vi "Configure Step Mode.vi"(0 "VISA resource name":refnum<visa-resource-name>, 1 "Step Frequency (50 Hz)":dbl=50.0 min=43.0 max=1200.0 format="%.2g", 2 "Step Voltage":T1 {"DC Voltage Step Level (0 V)" format="%.3g"; "AC Voltage Step Level (0 V)" format="%.3g"; "DC Voltage (0 V)" format="%.3g"; "AC Voltage (0 V)" format="%.3g"}, 5 "Frequency Step Level (0 Hz)":dbl format="%.1f", 7 "Step Time (1 s)":u32=1 min=1 max=100000, 9 "Step Count (1)":u32=1 min=1 max=99, 11 "error in (no error)":errorcluster, 12 "Step Sync (0: Immediate)":i32(ring) items=["Immediate", "Phase"], 13 "Step Phase (0.0 degrees)":dbl min=0.0 max=359.7 format="%.1f") -> (4 "VISA resource name out":refnum<visa-resource-name>, 15 "error out":errorcluster)   [LabVIEW 2015, in "BK Precision 983X Series.lvlib"]
doc: "Configures all the parameters for step mode.\n\nNote: Run <b>Configure Output Mode.vi</b> first to set the instrument to Step Mode before running this vi."
uses:
  <instrlib>/BK Precision 983X Series/BK Precision 983X Series.lvlib
panel:
  # "degree"
  # "Hz"
  # "V"
  # "V"
  # "V"
  # "V"
  # "s"
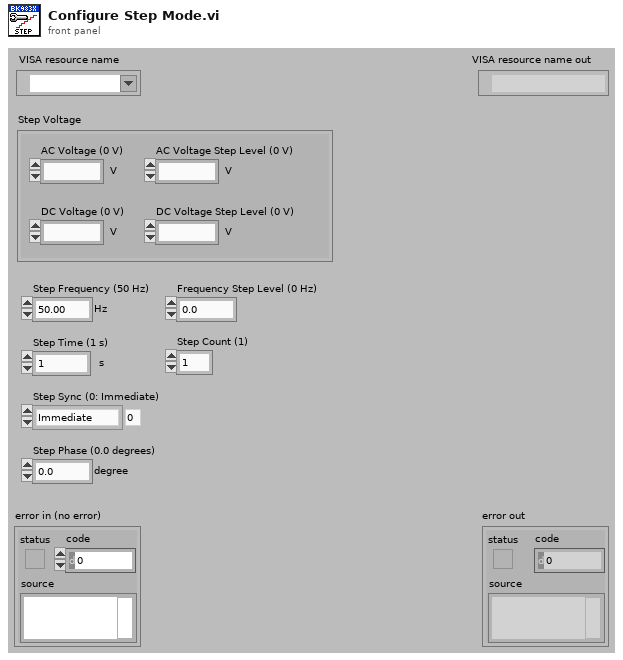
[diagram p1: front panel]
types:
  T1 = cluster{"AC Voltage (0 V)":dbl, "DC Voltage (0 V)":dbl, "AC Voltage Step Level (0 V)":dbl, "DC Voltage Step Level (0 V)":dbl}
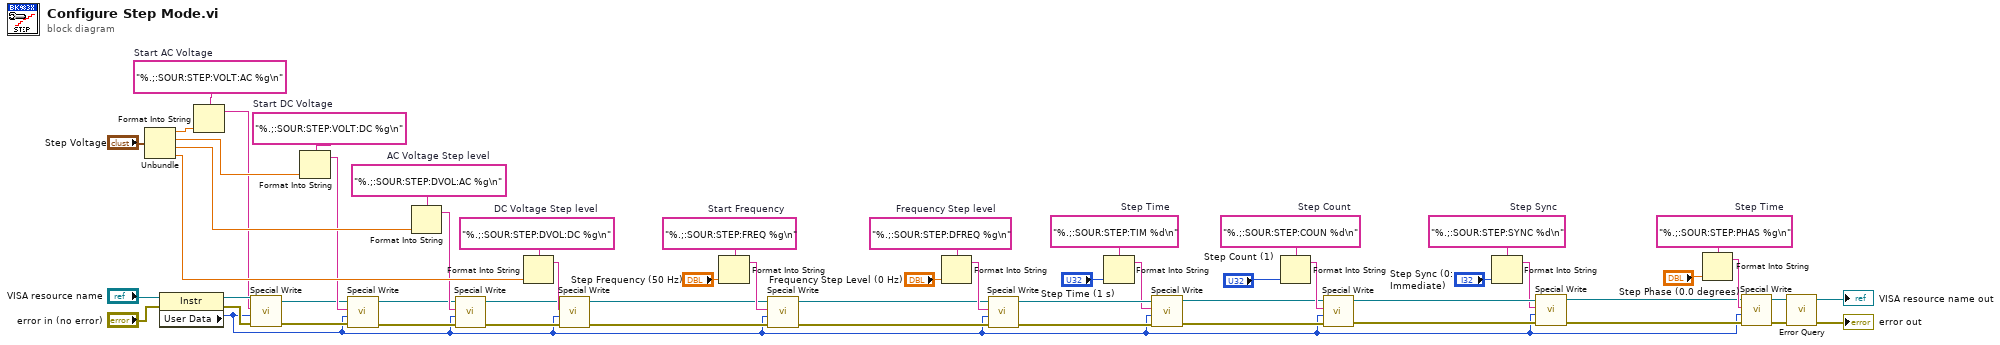
[diagram p0: block diagram]
diagram:
  w42 = "%.;:SOUR:STEP:SYNC %d\n"  # Step Sync
  w43 = "%.;:SOUR:STEP:COUN %d\n"  # Step Count
  w44 = "%.;:SOUR:STEP:TIM %d\n"  # Step Time
  w45 = "%.;:SOUR:STEP:DFREQ %g\n"  # Frequency Step level
  w46 = "%.;:SOUR:STEP:FREQ %g\n"  # Start Frequency
  w52 = "%.;:SOUR:STEP:DVOL:DC %g\n"  # DC Voltage Step level
  w53 = "%.;:SOUR:STEP:VOLT:DC %g\n"  # Start DC Voltage
  w54 = "%.;:SOUR:STEP:PHAS %g\n"  # Step Time
  w55 = "%.;:SOUR:STEP:DVOL:AC %g\n"  # AC Voltage Step level
  w56 = "%.;:SOUR:STEP:VOLT:AC %g\n"  # Start AC Voltage
  n1 = Unbundle("Step Voltage") -> ("AC Voltage (0 V)"=w50:dbl, "DC Voltage (0 V)"=w49:dbl, "AC Voltage Step Level (0 V)"=w48:dbl, "DC Voltage Step Level (0 V)"=w47:dbl)
  n2 = property class="Instr"(reference="VISA resource name", error in="error in (no error)") -> (reference out=w30:refnum<visa-resource-name>, error out=w29:errorcluster, "User Data"=w1:u32)
  n3 = Format Into String(format string=w56, w50) -> (resulting string=w28:string)  [unwired: 2 in, 1 out]
  n4 = call <instrlib>:"Special Write.vi"("error in (no error)"=w29, "Delay (0 ms)"=w1, "Input String"=w28, "VISA resource name"=w30) -> ("error out"=w25:errorcluster, "VISA resource name out"=w26:refnum<visa-resource-name>)  [unwired: 6 in]
  n5 = Format Into String(format string=w53, w49) -> (resulting string=w27:string)  [unwired: 2 in, 1 out]
  n6 = call <instrlib>:"Special Write.vi"("error in (no error)"=w25, "Delay (0 ms)"=w1, "Input String"=w27, "VISA resource name"=w26) -> ("error out"=w22:errorcluster, "VISA resource name out"=w23:refnum<visa-resource-name>)  [unwired: 6 in]
  n7 = Format Into String(format string=w55, w48) -> (resulting string=w24:string)  [unwired: 2 in, 1 out]
  n8 = call <instrlib>:"Special Write.vi"("error in (no error)"=w22, "Delay (0 ms)"=w1, "Input String"=w24, "VISA resource name"=w23) -> ("error out"=w19:errorcluster, "VISA resource name out"=w20:refnum<visa-resource-name>)  [unwired: 6 in]
  n9 = Format Into String(format string=w52, w47) -> (resulting string=w21:string)  [unwired: 2 in, 1 out]
  n10 = call <instrlib>:"Special Write.vi"("error in (no error)"=w19, "Delay (0 ms)"=w1, "Input String"=w21, "VISA resource name"=w20) -> ("error out"=w16:errorcluster, "VISA resource name out"=w17:refnum<visa-resource-name>)  [unwired: 6 in]
  n11 = Format Into String(format string=w46, "Step Frequency (50 Hz)") -> (resulting string=w18:string)  [unwired: 2 in, 1 out]
  n12 = call <instrlib>:"Special Write.vi"("error in (no error)"=w16, "Delay (0 ms)"=w1, "Input String"=w18, "VISA resource name"=w17) -> ("error out"=w13:errorcluster, "VISA resource name out"=w14:refnum<visa-resource-name>)  [unwired: 6 in]
  n13 = Format Into String(format string=w45, "Frequency Step Level (0 Hz)") -> (resulting string=w15:string)  [unwired: 2 in, 1 out]
  n14 = call <instrlib>:"Special Write.vi"("error in (no error)"=w13, "Delay (0 ms)"=w1, "Input String"=w15, "VISA resource name"=w14) -> ("error out"=w10:errorcluster, "VISA resource name out"=w12:refnum<visa-resource-name>)  [unwired: 6 in]
  n15 = Format Into String(format string=w44, "Step Time (1 s)") -> (resulting string=w11:string)  [unwired: 2 in, 1 out]
  n16 = call <instrlib>:"Special Write.vi"("error in (no error)"=w10, "Delay (0 ms)"=w1, "Input String"=w11, "VISA resource name"=w12) -> ("error out"=w7:errorcluster, "VISA resource name out"=w8:refnum<visa-resource-name>)  [unwired: 6 in]
  n17 = Format Into String(format string=w43, "Step Count (1)") -> (resulting string=w9:string)  [unwired: 2 in, 1 out]
  n18 = call <instrlib>:"Special Write.vi"("error in (no error)"=w7, "Delay (0 ms)"=w1, "Input String"=w9, "VISA resource name"=w8) -> ("error out"=w5:errorcluster, "VISA resource name out"=w6:refnum<visa-resource-name>)  [unwired: 6 in]
  n19 = Format Into String(format string=w42, "Step Sync (0: Immediate)") -> (resulting string=w4:string)  [unwired: 2 in, 1 out]
  n20 = call <instrlib>:"Special Write.vi"("error in (no error)"=w5, "Delay (0 ms)"=w1, "Input String"=w4, "VISA resource name"=w6) -> ("error out"=w2:errorcluster, "VISA resource name out"=w3:refnum<visa-resource-name>)  [unwired: 6 in]
  n21 = Format Into String(format string=w54, "Step Phase (0.0 degrees)") -> (resulting string=w33:string)  [unwired: 2 in, 1 out]
  n22 = call <instrlib>:"Special Write.vi"("error in (no error)"=w2, "Delay (0 ms)"=w1, "Input String"=w33, "VISA resource name"=w3) -> ("error out"=w34:errorcluster, "VISA resource name out"=w35:refnum<visa-resource-name>)  [unwired: 6 in]
  n23 = call <instrlib>:"Error Query.vi"("error in (no error)"=w34, "VISA resource name"=w35) -> ("error out"=→"error out":errorcluster, "VISA resource name out"=→"VISA resource name out":refnum<visa-resource-name>)  [unwired: 6 in, 2 out]
